vi "OutputMessageExample.vi"(5 "Sequence Context":refnum<k7>) -> (0 "error out":errorcluster)   [LabVIEW 2011]
doc: "Generates an output message every second for 10 seconds"
panel:
  # "This VI generates an output message every second for 10 seconds"
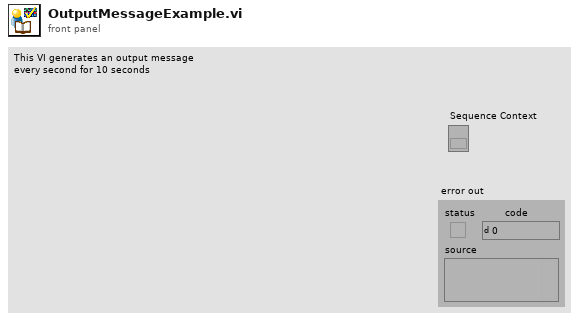
[diagram p1: front panel]
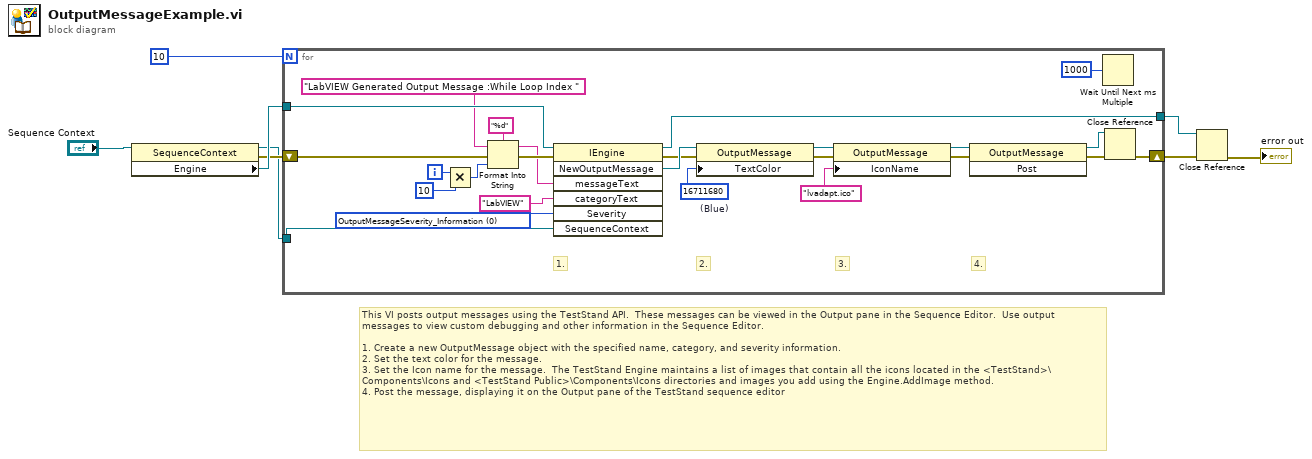
[diagram p0: block diagram]
diagram:
  # "This VI posts output messages using the TestStand API.  These messages can be viewed in the Output pane in the Sequence Editor.  Use output messages to view custom debugging and other information in the Sequence Editor.\n\n1. Create a new OutputMessage object with the specified name, category, and severity information.  \n2. Set the text color for the message.\n3. Set the Icon name for the message.  The TestStand Engine maintains a list of images that contain all the icons located in the <TestStand>\\Components\\Icons and <TestStand Public>\\Components\\Icons directories and images you add using the Engine.AddImage method. \n4. Post the message, displaying it on the Output pane of the TestStand sequence editor"
  n1 = property class="SequenceContext"(reference="Sequence Context") -> (reference out=w1:refnum<k7>, error out=w7:errorcluster, "Engine"=w8:refnum<k7>)  [unwired: 1 in]
  n2 = for {
    N: 10 -> [_]
    tunnel: w8 -> [w32]
    tunnel: w1 -> [w30]
    shift-right: [w14] -> w5
    shift-left: w7 -> [w31]
    tunnel: [w13] -> w3
    i -> [w12]
    w9 = u32 16711680  # (Blue)
    w24 = 0 items=["OutputMessageSeverity_Information", "OutputMessageSeverity_Warning", "OutputMessageSeverity_Error"] ("Severity")
    # "4."
    # "3."
    # "2."
    # "1."
    n3 = Multiply(x=w12, y=10) -> (x*y=w10:i32)
    n4 = Format Into String(format string="%d", initial string="LabVIEW Generated Output Message :While Loop Index ", error in=w31, w10) -> (resulting string=w26:string, error out=w27:errorcluster)
    n5 = invoke class="IEngine" method="NewOutputMessage"(reference=w32, error in=w27, "messageText"=w26, "categoryText"="LabVIEW", "Severity"=w24, "SequenceContext"=w30) -> (reference out=w13:refnum<k7>, error out=w22:errorcluster, "NewOutputMessage"=w23:refnum<k7>)  [unwired: 1 in, 4 out]
    n6 = property class="OutputMessage"(reference=w23, error in=w22, "TextColor"=w9) -> (reference out=w20:refnum<k7>, error out=w21:errorcluster)
    n7 = property class="OutputMessage"(reference=w20, error in=w21, "IconName"="lvadapt.ico") -> (reference out=w19:refnum<k7>, error out=w18:errorcluster)
    n8 = invoke class="OutputMessage" method="Post"(reference=w19, error in=w18) -> (reference out=w15:refnum<k7>, error out=w16:errorcluster)  [unwired: 1 in, 1 out]
    n9 = Wait Until Next ms Multiple(millisecond multiple=u32 1000) -> ()  [unwired: 1 out]
    n10 = Close Reference(reference=w15, error in (no error)=w16) -> (error out=w14:errorcluster)
  }
  n11 = Close Reference(reference=w3, error in (no error)=w5) -> (error out=→"error out":errorcluster)
